vi "MicroSlide-Initialize.vi"(0 "VISA resource name":refnum<visa-resource-name>="COM15") -> (4 "VRN OUT":refnum<visa-resource-name>="COM15", 15 "Error OUT":errorcluster)   [LabVIEW 2011]
uses:
  <vilib>/Instr/_visa.llb/VISA Configure Serial Port (Instr).vi
panel:
  out "Received Buffer":string
  out "HF Erreur":bool
  out "SI Erreur":bool
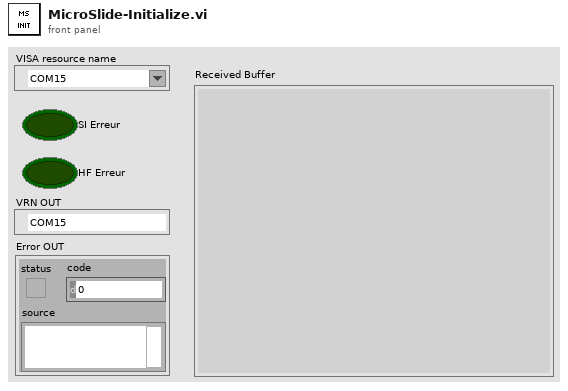
[diagram p1: front panel]
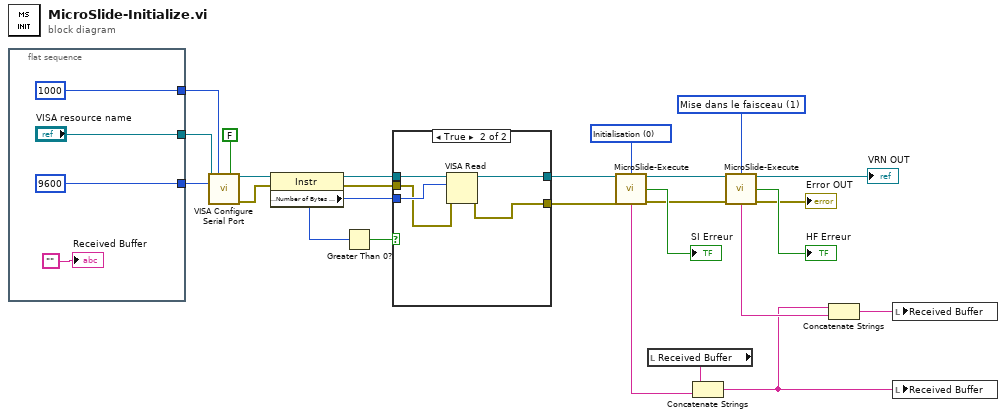
[diagram p0: block diagram]
diagram:
  w18 = u16 1 items=["Initialisation", "Mise dans le faisceau", "Retirer du faisceau"] ("Commande")
  w22 = u16 0 items=["Initialisation", "Mise dans le faisceau", "Retirer du faisceau"] ("Commande")
  n1 = flat-sequence {
    tunnel: ["VISA resource name"] -> w24
    tunnel: [u32 9600 ("Baud Rate")] -> w23
    tunnel: [u32 1000 ("timeout (10sec)")] -> w14
    frame #0 {
      "Received Buffer" <- ""
    }
  }
  n2 = call-poly "VISA Configure Serial Port"("VISA resource name"=w24, "timeout (10sec)"=w14, "Enable Termination\nChar (T)"=FALSE ("Enable Termination\nChar (T)"), "baud rate (9600)"=w23) -> ("VISA resource name out"=w13:refnum<visa-resource-name>, "error out"=w12:errorcluster)  [unwired: 10 in]
  n3 = property class="Instr"(reference=w13, error in=w12) -> (reference out=w10:refnum<visa-resource-name>, error out=w8:errorcluster, "Serial Settings:Number of Bytes at Serial Port"=w9:u32)
  n4 = Greater Than 0?(x=w9) -> (x > 0?=w11:bool)
  n5 = case shown="True" w11 {
    tunnel: w10 -> [w31 w36]
    tunnel: w9 -> [_ w35]
    tunnel: w8 -> [w30 w34]
    tunnel: [w30 w33] -> w7
    tunnel: [w31 w32] -> w6
    frame False {
    }
    frame True {
      n6 = VISA Read(VISA resource name=w36, byte count=w35, error in (no error)=w34) -> (VISA resource name out=w32:refnum<visa-resource-name>, error out=w33:errorcluster)  [unwired: 2 out]
    }
  }
  n7 = call "MicroSlide-Execute.vi"("VISA resource name"=w6, "Commande"=w22, "Error IN"=w7) -> ("VRN OUT"=w20:refnum<visa-resource-name>, "Erreur"=→"SI Erreur":bool, "Received Buffer"=w5:string, "Error OUT"=w19:errorcluster)  [unwired: 9 in]
  n8 = local read "Received Buffer"() -> (w4:string)
  n9 = Concatenate Strings(w4, w5) -> (w1:string)
  n10 = call "MicroSlide-Execute.vi"("VISA resource name"=w20, "Commande"=w18, "Error IN"=w19) -> ("VRN OUT"=→"VRN OUT":refnum<visa-resource-name>, "Erreur"=→"HF Erreur":bool, "Received Buffer"=w2:string, "Error OUT"=→"Error OUT":errorcluster)  [unwired: 9 in]
  n11 = Concatenate Strings(w1, w2) -> (w3:string)
  n12 = local write "Received Buffer"(w3) -> ()
  n13 = local write "Received Buffer"(w1) -> ()
